vi "Process Auto-Sequence.vi"(7 "Data Cluster In":T1, 8 "error in":errorcluster, 11 "y":dbl) -> (0 "error out":errorcluster, 2 "Again Process?":bool, 5 "Data Cluster Out":T1)   [LabVIEW 2021, in "RT-AutoSequence.lvlib"]
uses:
  RT-AutoSequence.lvlib
  Module Data--cluster.ctl
  TCP Engine/Controls/TCP Engine I&O  Interupt Cluster.ctl
  Digital Output/Controls/DO Update Cluster.ctl
  8096dcf1-40de-4ee2-9ef8-c92b8b4be91c.vi
  <userlib>/_OpenG.lib/array/array.llb/Search 1D Array (DBL)__ogtk.vi
  <userlib>/_OpenG.lib/array/array.llb/Index 1D Array Elements (Boolean)__ogtk.vi
  <userlib>/_OpenG.lib/array/array.llb/Index 1D Array Elements (String)__ogtk.vi
  <userlib>/_OpenG.lib/array/array.llb/Delete Elements from 1D Array (String)__ogtk.vi
  <userlib>/_OpenG.lib/array/array.llb/Delete Elements from 1D Array (Boolean)__ogtk.vi
  <userlib>/_OpenG.lib/array/array.llb/Delete Elements from 1D Array (DBL)__ogtk.vi
  <userlib>/_OpenG.lib/array/array.llb/openg_array.lvlib
  TCP Engine/TCP Engine.lvlib
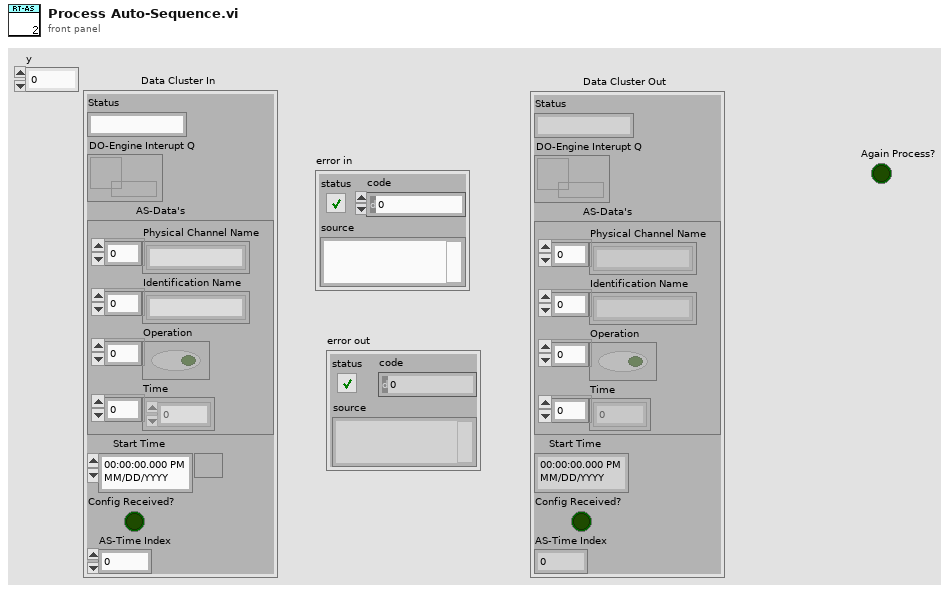
[diagram p1: front panel]
types:
  T1 = typedef "RT-AutoSequence.lvlib/Module Data--cluster.ctl" = cluster{"Status":string, "DO-Engine Interupt Q":refnum<queue>, "AS-Data's":cluster{"Physical Channel Name":string[], "Identification Name":string[], "Operation":bool[], "Time":dbl[]}, "Start Time":timestamp, "Config Received?":bool, "AS-Time Index":i32}
  T2 = typedef "DO Update Cluster.ctl" = cluster{"Channel":string[], "Data":u8[]}
  T3 = typedef "TCP Engine.lvlib/TCP Engine I&O  Interupt Cluster.ctl" = cluster{" Stop":bool, "JSON Variant":variant}
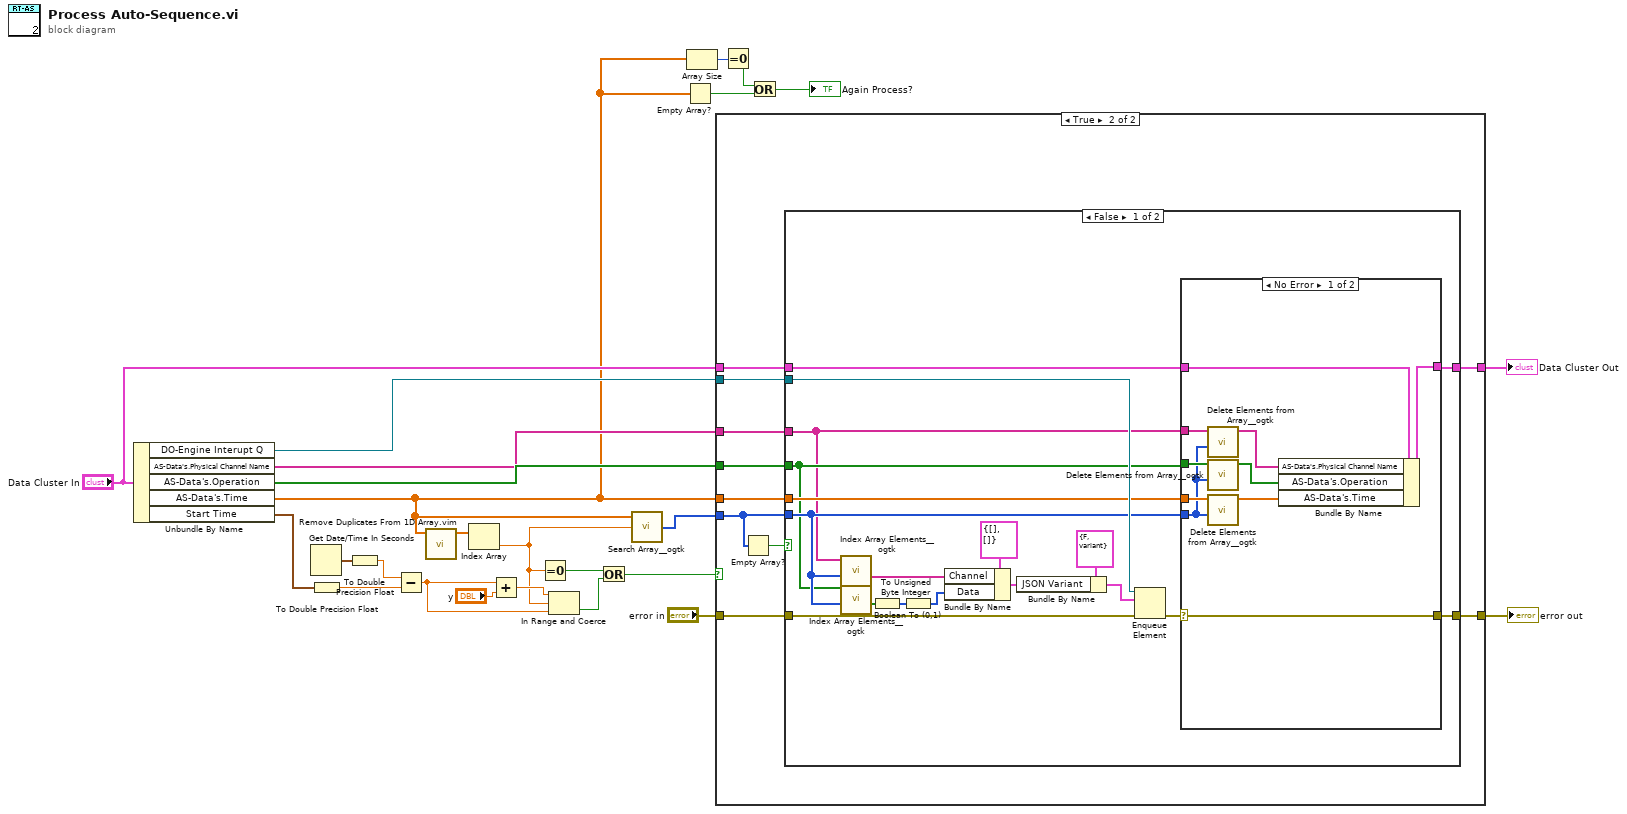
[diagram p0: block diagram]
diagram:
  n1 = Unbundle By Name("Data Cluster In") -> ("DO-Engine Interupt Q"=w17:refnum<queue>, "AS-Data's.Physical Channel Name"=w18:string[], "AS-Data's.Operation"=w19:bool[], "AS-Data's.Time"=w11:dbl[], "Start Time"=w20:timestamp)
  n2 = Get Date/Time In Seconds() -> (seconds since 1Jan1904=w25:timestamp)
  n3 = To Double Precision Float(number=w20) -> (double precision float=w23:dbl)
  n4 = To Double Precision Float(number=w25) -> (double precision float=w24:dbl)
  n5 = Subtract(x=w24, y=w23) -> (x-y=w2:dbl)
  n6 = call "Remove Duplicates From 1D Array.vim"("array"=w11) -> ("array with duplicates removed"=w14:dbl[])  [unwired: 10 in]
  n7 = Index Array(array=w14) -> (element=w3:dbl)  [unwired: 1 in]
  n8 = Add(x=w2, y="y") -> (x+y=w5:dbl)
  n9 = Equal To 0?(x=w3) -> (x = 0?=w7:bool)
  n10 = In Range and Coerce(upper limit=w5, x=w3, lower limit=w2) -> (In Range?=w1:bool)  [unwired: 1 out]
  n11 = Or(x=w7, y=w1) -> (x .or. y?=w6:bool)
  n12 = call-poly <userlib>:"Search Array__ogtk.vi"("Array"=w11, "Element Data"=w3) -> ("Indices of Elements"=w13:i32[])  [unwired: 7 in]
  n13 = Empty Array?(array=w11) -> (empty?=w12:bool)
  n14 = Array Size(array=w11) -> (size(s)=w10:i32)
  n15 = case shown="True" w6 {
    tunnel: "error in" -> [w26 w37]
    tunnel: [w26 w35] -> w21
    tunnel: w19 -> [_ w34]
    tunnel: w18 -> [_ w33]
    tunnel: w17 -> [_ w32]
    tunnel: [w27 w31] -> w16
    tunnel: "Data Cluster In" -> [w27 w30]
    tunnel: w11 -> [_ w29]
    tunnel: w13 -> [_ w28]
    frame False {
    }
    frame True {
      n16 = Empty Array?(array=w28) -> (empty?=w36:bool)
      n17 = case shown="False" w36 {
        tunnel: [w40 w68] -> w35
        tunnel: w37 -> [w46 w68]
        tunnel: w28 -> [w45 _]
        tunnel: w34 -> [w39 _]
        tunnel: w33 -> [w38 _]
        tunnel: w32 -> [w47 _]
        tunnel: [w42 w67] -> w31
        tunnel: w30 -> [w43 w67]
        tunnel: w29 -> [w44 _]
        frame False {
          n18 = call-poly <userlib>:"Index Array Elements__ogtk.vi"("indices"=w45, "array"=w38) -> ("elements"=w52:string[])  [unwired: 9 in]
          n19 = call-poly <userlib>:"Index Array Elements__ogtk.vi"("indices"=w45, "array"=w39) -> ("elements"=w51:bool[])  [unwired: 9 in]
          n20 = Boolean To (0,1)(Boolean=w51) -> (0, 1=w50:i16[])
          n21 = To Unsigned Byte Integer(number=w50) -> (unsigned 8bit integer=w49:u8[])
          n22 = Bundle By Name(cluster=T2 {"Channel"=[], "Data"=[]} ("DO Update Cluster"), "Channel"=w52, "Data"=w49) -> (w48:T2)
          n23 = Bundle By Name(cluster=T3 {" Stop"=FALSE, "JSON Variant"=variant(string "")} ("I/O  Interupt Cluster"), "JSON Variant"=w48) -> (w55:T3)
          n24 = Enqueue Element(queue=w47, element=w55, error in (no error)=w46) -> (error out=w41:errorcluster)  [unwired: 1 in, 2 out]
          n25 = case shown="No Error" w41 {
            selector: w41 -> [w63 _]
            tunnel: w45 -> [w57 _]
            tunnel: w44 -> [w62 _]
            tunnel: w43 -> [w65 w66]
            tunnel: [w64 w66] -> w42
            tunnel: [w63 _] -> w40
            tunnel: w39 -> [w60 _]
            tunnel: w38 -> [w59 _]
            frame No Error {
              n26 = call-poly <userlib>:"Delete Elements from Array__ogtk.vi"("indices"=w57, "array"=w59) -> ("array w/ subset deleted"=w56:string[])  [unwired: 8 in, 1 out]
              n27 = call-poly <userlib>:"Delete Elements from Array__ogtk.vi"("indices"=w57, "array"=w60) -> ("array w/ subset deleted"=w58:bool[])  [unwired: 8 in, 1 out]
              n28 = call-poly <userlib>:"Delete Elements from Array__ogtk.vi"("indices"=w57, "array"=w62) -> ("array w/ subset deleted"=w61:dbl[])  [unwired: 8 in, 1 out]
              n29 = Bundle By Name(cluster=w65, "AS-Data's.Physical Channel Name"=w56, "AS-Data's.Operation"=w58, "AS-Data's.Time"=w61) -> (w64:T1)
            }
            frame Error {
            }
          }
        }
        frame True {
        }
      }
    }
  }
  "Data Cluster Out" <- w16
  "error out" <- w21
  n30 = Equal To 0?(x=w10) -> (x = 0?=w9:bool)
  n31 = Or(x=w9, y=w12) -> (x .or. y?=→"Again Process?":bool)
